vi "GrabToTrackerFastLoop.vi"(0 "IMAQ Refnum in":refnum<k11>, 2 "ResultManager":T3, 3 "QTrk Instance":T4, 4 "ROIs":cluster{"X":i32, "Y":i32}[](array[cluster]), 6 "stop":refnum<vi>, 9 "#ROI":u32, 13 "ROI Size":cluster{"X":i32, "Y":i32}) -> ()   [LabVIEW 2011]
uses:
  qtrk/QTrkLVBinding/QTrkInstance.ctl
  qtrk/QTrkLVBinding/ResultManagerInstance.ctl
  Main/Motors/MotorPosType.ctl
  Main/Typedefs/XYf.ctl
  qtrk/QTrkLVBinding/QTrkLocalizationJob.ctl
  qtrk/QTrkLVBinding/XYZf.ctl
  qtrk/QTrkLVBinding/QTrkPixelDataType.ctl
  qtrk/QTrkLVBinding/QTrkDLL.vi
  Main/GlobalVariables.vi
panel:
  out "stop local":bool
  out "Current Position":T1
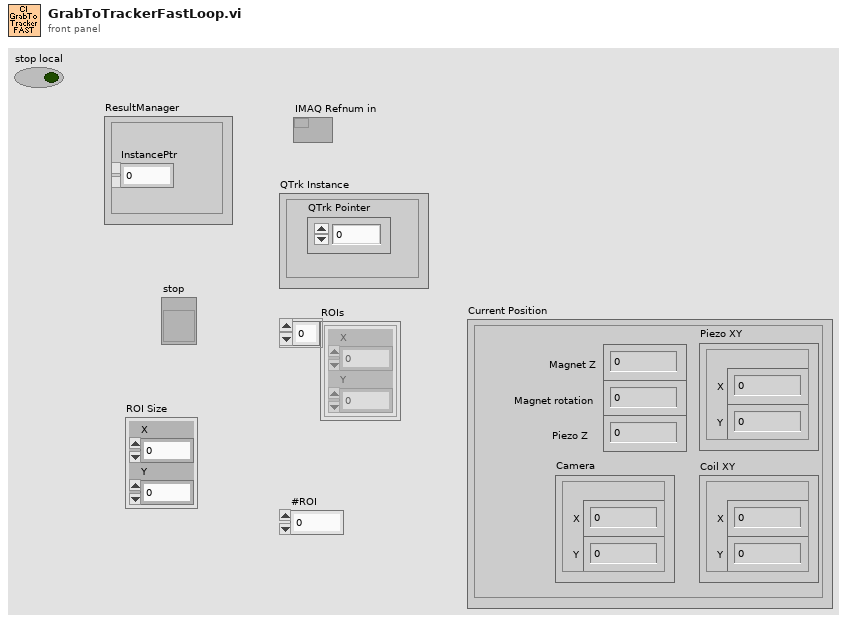
[diagram p1: front panel]
types:
  T1 = typedef "MotorPosType.ctl" = cluster{"Magnet Z":dbl, "Magnet rotation":dbl, "Camera":T2, "Piezo XY":T2, "Piezo Z":dbl, "Coil XY":T2}
  T2 = typedef "XYf.ctl" = cluster{"X":sgl, "Y":sgl}
  T3 = typedef "ResultManagerInstance.ctl" = cluster{"InstancePtr":u64}
  T4 = typedef "QTrkInstance.ctl" = cluster{"QTrk Pointer":u64}
  T5 = typedef "MotorStateType.ctl" = cluster{"Enabled?":bool, "Current Position":T1, "Update counter":i32}
  T6 = typedef "IMAQ Image.ctl" = refnum<image>
  T7 = typedef "QTrkPixelDataType.ctl" = enum16{"QTrkU8", "QTrkU16", "QTrkFloat"}
  T8 = enum32{"Map Pixel Pointer", "Unmap Pixel Pointer", "Get Pixels Infos"}
  T9 = typedef "QTrkLocalizationJob.ctl" = cluster{"Frame#":u32, "Timestamp":u32, "ZLUT Index / bead#":i32, "Initial guess":T10}
  T10 = typedef "XYZf.ctl" = cluster{"X":sgl, "Y":sgl, "Z":sgl}
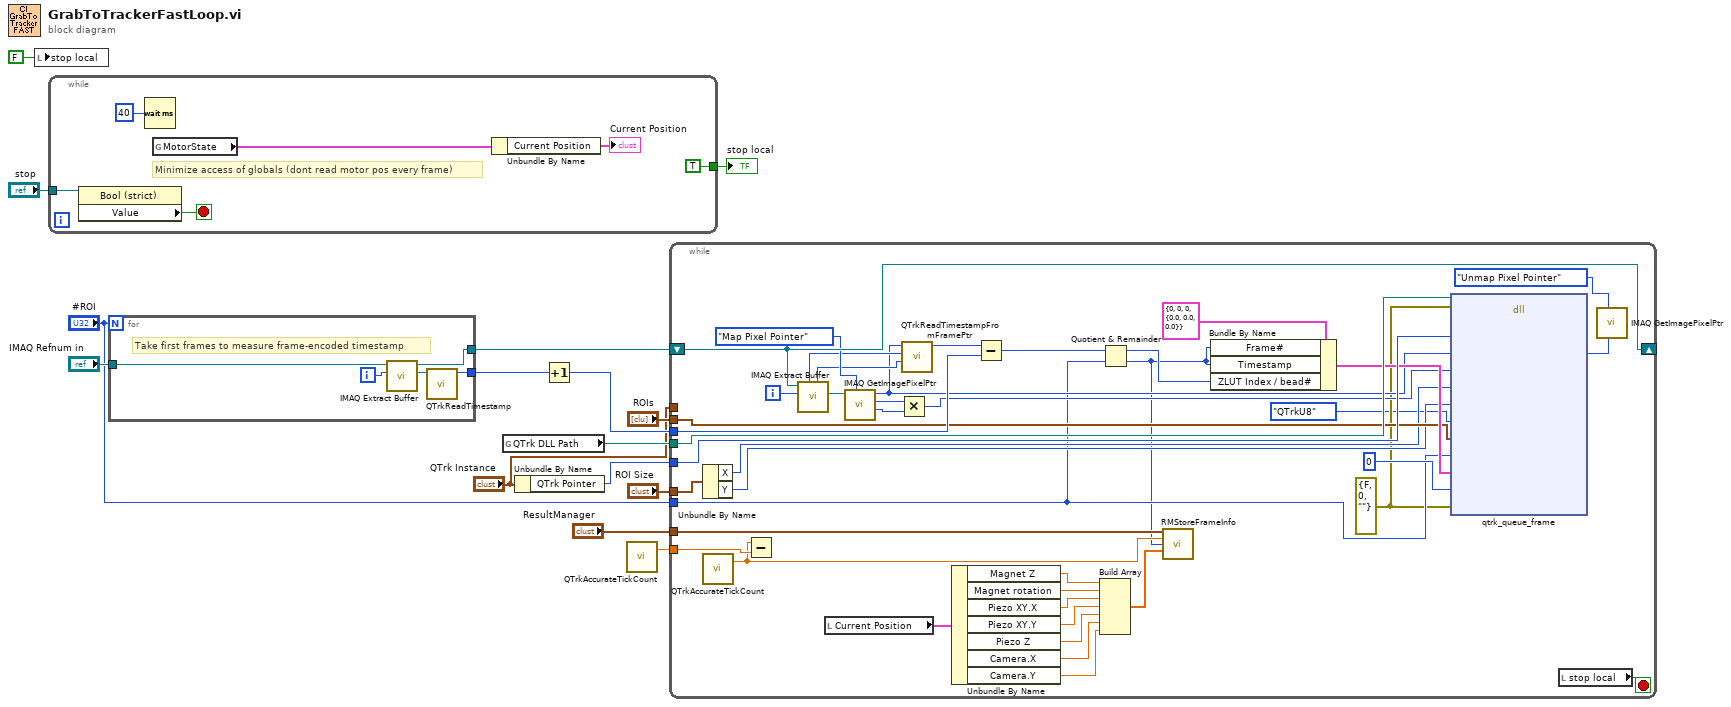
[diagram p0: block diagram]
diagram:
  n1 = local write "stop local"(FALSE ("stop local")) -> ()
  n2 = while {
    tunnel: "stop" -> [w18]
    tunnel: [TRUE ("stop local")] -> w3
    stop <- w17 stop-if-true
    # "Minimize access of globals (dont read motor pos every frame)"
    n3 = property on="Property Node" class="Bool (strict)"(reference=w18) -> ("Value"=w17:bool)  [unwired: 1 in, 2 out]
    n4 = Wait (ms)(milliseconds to wait=u32 40) -> ()  [unwired: 1 out]
    n5 = global read "GlobalVariables.vi" "MotorState"() -> (w21:T5)
    n6 = Unbundle By Name(w21) -> ("Current Position"=→"Current Position":T1)
  }
  "stop local" <- w3
  n7 = for {
    N: "#ROI" -> [_]
    tunnel: "IMAQ Refnum in" -> [w25]
    tunnel: [w24] -> w10
    tunnel: [w22] -> w12
    i -> [w23]
    # "Take first frames to measure frame-encoded timestamp"
    n8 = call <vilib>:"IMAQ Extract Buffer.vi"("Buffer to extract"=w23, "IMAQ Session In"=w25) -> ("Image Out"=w26:T6, "IMAQ Session Out"=w24:refnum<k11>)  [unwired: 4 in, 4 out]
    n9 = call "QTrkReadTimestamp.vi"("Image"=w26) -> ("timestamp"=w22:u32)  [unwired: 10 in]
  }
  n10 = global read "QTrkDLL.vi" "QTrk DLL Path"() -> (w7:path)
  n11 = Unbundle By Name("QTrk Instance") -> ("QTrk Pointer"=w5:u64)
  n12 = Increment(x=w12) -> (x+1=w9:u32)
  n13 = call "QTrkAccurateTickCount.vi"() -> ("tick count (ms)"=w13:dbl)  [unwired: 2 in, 1 out]
  n14 = while {
    shift-right: [w68] -> _
    shift-left: w10 -> [w68]
    tunnel: "QTrk Instance" -> [_]
    tunnel: w13 -> [w67]
    tunnel: "ROIs" -> [w40]
    tunnel: w9 -> [w66]
    tunnel: "ROI Size" -> [w65]
    tunnel: "#ROI" -> [w33]
    tunnel: w7 -> [w62]
    tunnel: w5 -> [w61]
    tunnel: "ResultManager" -> [w53]
    i -> [w63]
    stop <- w27 stop-if-true
    w32 = errorcluster {"status"=FALSE, "code"=0, "source"=""} ("err")
    n15 = Unbundle By Name(w65) -> ("X"=w39:i32, "Y"=w38:i32)
    n16 = call "QTrkAccurateTickCount.vi"() -> ("tick count (ms)"=w52:dbl)  [unwired: 2 in, 1 out]
    n17 = Subtract(x=w52, y=w67) -> ()  [unwired: 1 out]
    n18 = call <vilib>:"IMAQ Extract Buffer.vi"("Buffer to extract"=w63, "IMAQ Session In"=w68) -> ("Image Out"=w51:T6, "Actual Height"=w44:u32, "Actual Width"=w45:u32)  [unwired: 4 in, 3 out]
    n19 = local read "Current Position"() -> (w54:T1)
    n20 = call "IMAQ GetImagePixelPtr"("Function"=T8."Map Pixel Pointer", "Image"=w51) -> ("Pixel Size (Bytes)"=w35:i32, "LineWidth(Pixels)"=w36:i32, "Pixel Pointer out"=w43:u64)  [unwired: 4 in, 3 out]
    n21 = Multiply(x=w36, y=w35) -> (x*y=w34:i32)
    n22 = call "QTrkReadTimestampFromFramePtr.vi"("height"=w44, "width"=w45, "imageptr"=w43) -> ("timestamp"=w42:u32)  [unwired: 8 in]
    n23 = Unbundle By Name(w54) -> ("Magnet Z"=w60:dbl, "Magnet rotation"=w59:dbl, "Piezo XY.X"=w58:sgl, "Piezo XY.Y"=w57:sgl, "Piezo Z"=w55:dbl, "Camera.X"=w31:sgl, "Camera.Y"=w30:sgl)
    n24 = Subtract(x=w42, y=w66) -> (x-y=w64:u32)
    n25 = Build Array(w60, w59, w58, w57, w55, w31, w30) -> (w56:dbl[])
    n26 = Quotient & Remainder(x=w64, y=w33) -> (x-y*floor(x/y)=w37:u32, floor(x/y)=w29:u32)
    n27 = call "RMStoreFrameInfo.vi"("ResultManager"=w53, "timestamp"=w52, "frame"=w29, "columns"=w56) -> ()  [unwired: 10 in, 2 out]
    n28 = Bundle By Name(cluster=T9 {"Frame#"=0, "Timestamp"=0, "ZLUT Index / bead#"=0, "Initial guess"={"X"=0.0, "Y"=0.0, "Z"=0.0}} ("Queue Params"), "Frame#"=w29, "Timestamp"=w29, "ZLUT Index / bead#"=w37) -> (w46:T9)
    n29 = dll-call lib="D:/jcnossen1/cudaqi-tracker/bin/jtrk-labview.dll" fn="qtrk_queue_frame"(path in=w62, error in=w32, "tracker"=w61, "image"=w43, "pitch"=w34, "width"=w39, "height"=w38, "pixelFormat"=QTrkPixelDataType."QTrkU8" ("Pixel data type"), "positions"=w40, "numROI"=w33, "jobInfo"=w46, "flags"=0, "err"=w32) -> ("image"=w48:u64)  [unwired: 12 in, 2 out]
    n30 = local read "stop local"() -> (w27:bool)
    n31 = call "IMAQ GetImagePixelPtr"("Pixel Pointer in"=w48, "Function"=T8."Unmap Pixel Pointer") -> ()  [unwired: 4 in, 6 out]
  }
